vi "参数选择.vi"(11 "项名":string[](array[string])) -> (3 "字符串":string)   [LabVIEW 2016, in "下拉列表.xctl"]
panel:
  in  "列表框":T1
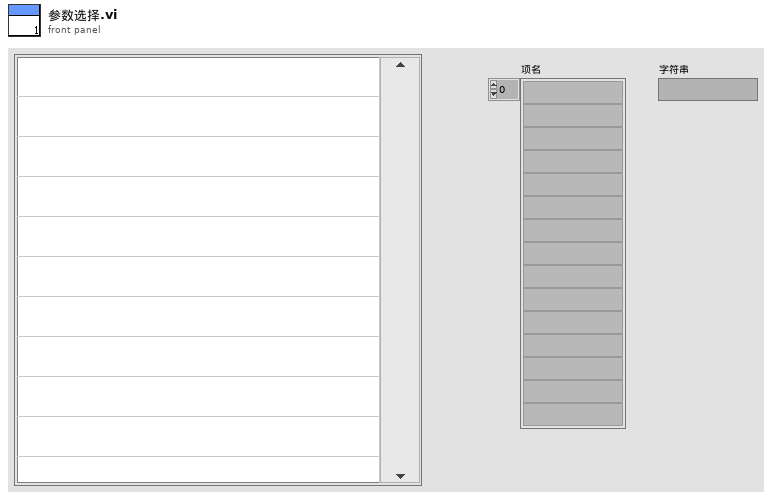
[diagram p1: front panel]
types:
  T1 = typedef "下拉列表.xctl/列表框.ctl" = i32
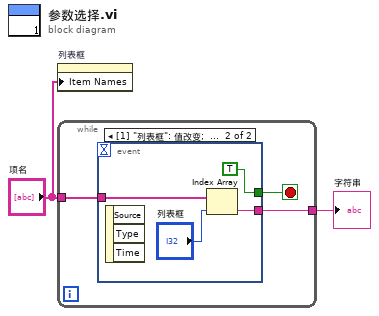
[diagram p0: block diagram]
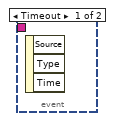
[diagram p2: hidden frame]
diagram:
  n1 = property on="列表框" class="LstBox (严格)"("Item Names"="项名") -> ()  [unwired: 2 in, 2 out]
  n2 = while {
    tunnel: "项名" -> [w5]
    tunnel: [w4] -> w1
    stop <- w3 stop-if-true
    n3 = event shown="[1] \"列表框\": 值改变;  前面板关闭" {
      selector: _ -> [_ _]
      dyn-events: _ -> [_ _]
      timeout: _ -> [_ _]
      tunnel: w5 -> [_ w9]
      tunnel: [_ w7] -> w4
      tunnel: [_ TRUE] -> w3
      event Timeout {
        n4 = event-data() -> ()  [unwired: 1 in, 3 out]
      }
      event Value Change; Panel Close {
        n5 = event-data() -> ()  [unwired: 1 in, 3 out]
        n6 = Index Array(array=w9, index="列表框") -> (element=w7:string)
      }
    }
  }
  "字符串" <- w1
